vi "get FW Version Number LV.vi"(11 "instance":i32) -> (3 "function return":dbl)   [LabVIEW 2023, in "SADI_FW3.lvlib"]
doc: "SADI_API_Wrapper double getFWVersionNumber_LV(int instance);\nSADI_API_Wrapper float getFWVersionNumber_LV(int instance);"
uses:
  SADI_FW3.lvlib
  SADI_FW3.dll
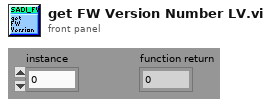
[diagram p1: front panel]
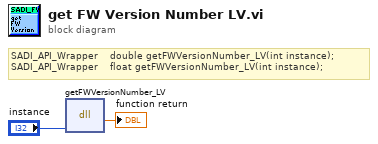
[diagram p0: block diagram]
diagram:
  # "SADI_API_Wrapper    double getFWVersionNumber_LV(int instance);\nSADI_API_Wrapper    float getFWVersionNumber_LV(int instance);"
  n1 = dll-call lib="C:/Users/loran/Documents/School/24_Spring/Controls Lab/EML4314c_Sp24_framework_0/LVLib/SADI_FW3.*" fn="getFWVersionNumber_LV"("instance"="instance") -> (→"function return":dbl)  [unwired: 4 in, 2 out]
